vi "RearrangePoints.vi"() -> (2 "Iterations":i32)   [LabVIEW 2010]
panel:
  out "error out":errorcluster
  in  "error in (no error)":errorcluster
  in  "Parameters":T1={"number of planes"=4, "z step"=1.9999999999999998e-05, "pixel dwell time"=1.0000000000000001e-11, "z frequency"=10.0, "number of pixels"=100, "smooth points"=10, "smooth line"=10, "Sine\nSawtooth"=FALSE, "PointSorting"=0, "Sort Points"=FALSE, "X-pixels"=256.0, "Y-lines"=256.0} {"Y-lines" min=1 step=1; "X-pixels" min=1 step=1; "PointSorting" items=["No Difference", "Every Second Point", "Down / Up"]; "smooth line" min=1; "smooth points" min=1; "number of pixels" min=1; "z frequency" format="%_4g"; "number of planes" min=1}
  out "XYZ Point coordinates updated (pixels) Up":dbl[][](array[numeric])
  out "XYZ Point coordinates updated (pixels) Down":dbl[][](array[numeric])
  in  "XYZ Point coordinates (pixels)":dbl[][](array[numeric])
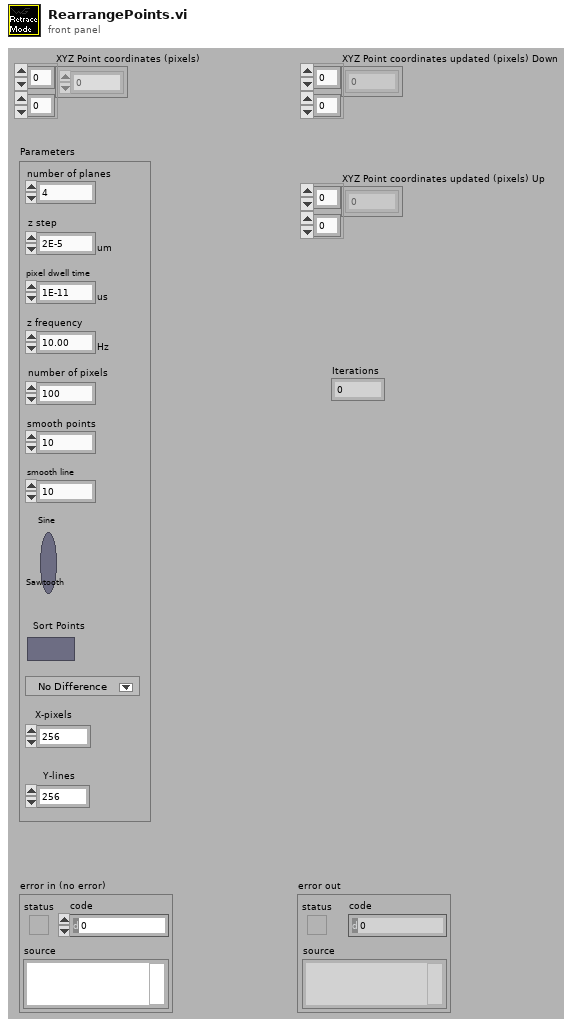
[diagram p1: front panel]
types:
  T1 = cluster{"number of planes":i32, "z step":dbl[unit], "pixel dwell time":dbl[unit], "z frequency":dbl[unit], "number of pixels":i32, "smooth points":i32, "smooth line":i32, "Sine\nSawtooth":bool, "PointSorting":u16, "Sort Points":bool, "X-pixels":sgl, "Y-lines":sgl}
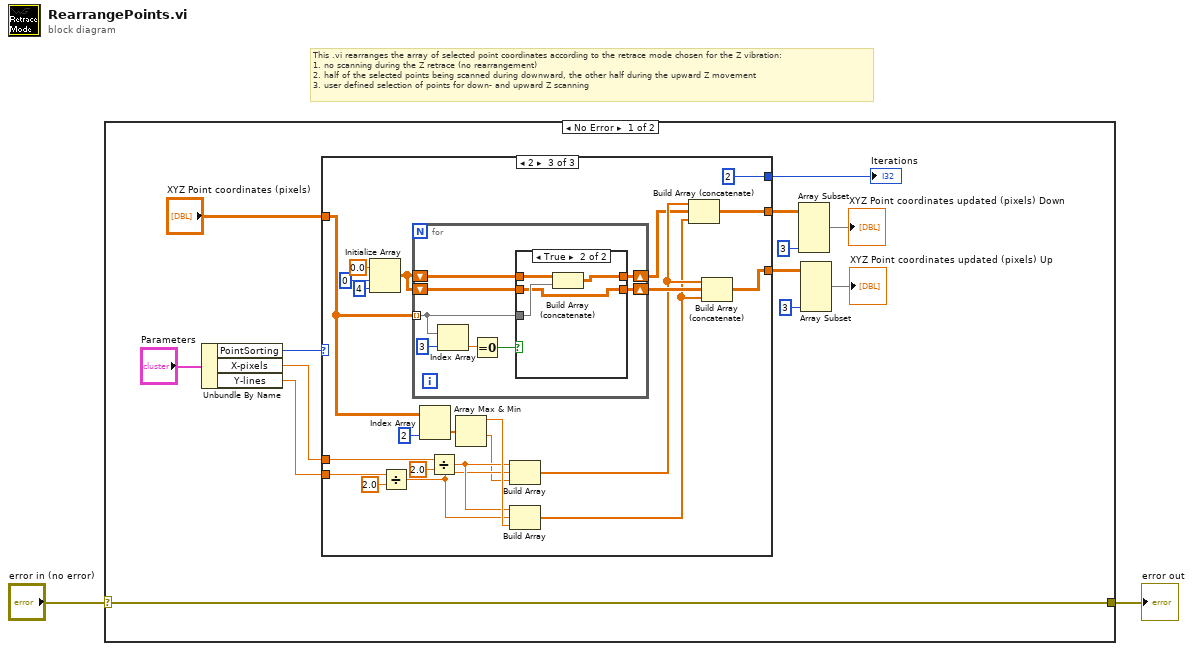
[diagram p0: block diagram]
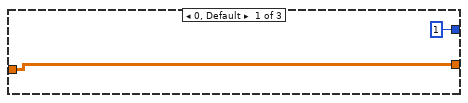
[diagram p2: hidden frame]
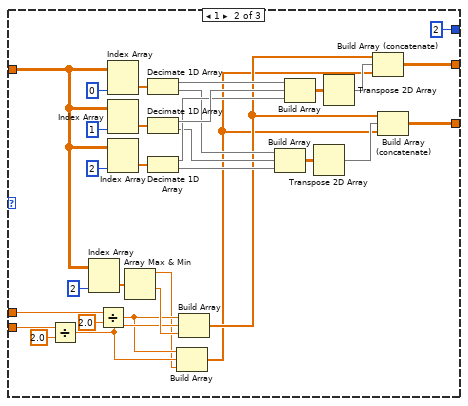
[diagram p3: hidden frame]
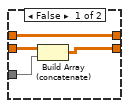
[diagram p4: hidden frame]
diagram:
  # "This .vi rearranges the array of selected point coordinates according to the retrace mode chosen for the Z vibration:\n1. no scanning during the Z retrace (no rearrangement)\n2. half of the selected points being scanned during downward, the other half during the upward Z movement\n3. user defined selection of points for down- and upward Z scanning"
  n1 = case shown="No Error" "error in (no error)" {
    selector: "error in (no error)" -> [w3 w88]
    tunnel: [w3 w88] -> w1
    frame No Error {
      n2 = Unbundle By Name("Parameters") -> ("PointSorting"=w6:u16, "X-pixels"=w5:sgl, "Y-lines"=w4:sgl)
      n3 = case shown="2" w6 {
        tunnel: "XYZ Point coordinates (pixels)" -> [w17 w23 w58]
        tunnel: w5 -> [_ w22 w60]
        tunnel: w4 -> [_ w21 w59]
        tunnel: [w17 w20 w57] -> w13
        tunnel: [_ w19 w53] -> w11
        tunnel: [1 2 2] -> w15
        frame 0, Default {
        }
        frame 1 {
          n4 = Divide(x=w21, y=2.0) -> (x/y=w28:dbl)
          n5 = Index Array(array=w23, index (col)=2 ("disabled index (col)")) -> (element=w32:dbl[])  [unwired: 1 in]
          n6 = Divide(x=w22, y=2.0) -> (x/y=w27:dbl)
          n7 = Index Array(array=w23, index (col)=0 ("disabled index (col)")) -> (element=w46:dbl[])  [unwired: 1 in]
          n8 = Index Array(array=w23, index (col)=1 ("disabled index (col)")) -> (element=w45:dbl[])  [unwired: 1 in]
          n9 = Index Array(array=w23, index (col)=2 ("disabled index (col)")) -> (element=w44:dbl[])  [unwired: 1 in]
          n10 = Array Max & Min(array=w32) -> (max value=w26:dbl, min value=w29:dbl)  [unwired: 2 out]
          n11 = Decimate 1D Array(w46) -> (w42:dbl[], w36:dbl[])
          n12 = Decimate 1D Array(w45) -> (w41:dbl[], w37:dbl[])
          n13 = Decimate 1D Array(w44) -> (w40:dbl[], w38:dbl[])
          n14 = Build Array(w27, w28, w26) -> (w24:dbl[])
          n15 = Build Array(w27, w28, w29) -> (w25:dbl[])
          n16 = Build Array(w36, w37, w38) -> (w39:dbl[][])
          n17 = Build Array(w42, w41, w40) -> (w43:dbl[][])
          n18 = Transpose 2D Array(2D array=w39) -> (transposed array=w34:dbl[][])
          n19 = Transpose 2D Array(2D array=w43) -> (transposed array=w35:dbl[][])
          n20 = Build Array (concatenate)(w25, w35, w24) -> (w20:dbl[][])
          n21 = Build Array (concatenate)(w25, w34, w24) -> (w19:dbl[][])
        }
        frame 2 {
          n22 = Initialize Array(0.0 ("element"), 0 ("dimension size"), 4 ("dimension size")) -> (w69:dbl[][])
          n23 = Divide(x=w59, y=2.0) -> (x/y=w66:dbl)
          n24 = for {
            tunnel: w58 -> [w76] mode=indexing
            shift-right: [w74] -> w52
            shift-left: w69 -> [w75]
            shift-right: [w72] -> w56
            shift-left: w69 -> [w73]
            n25 = Index Array(array=w76, index=3) -> (element=w78:dbl)
            n26 = Equal To 0?(x=w78) -> (x = 0?=w77:bool)
            n27 = case shown="True" w77 {
              tunnel: w76 -> [w80 w86]
              tunnel: w75 -> [w83 w87]
              tunnel: [w83 w85] -> w74
              tunnel: w73 -> [w82 w84]
              tunnel: [w81 w84] -> w72
              frame False {
                n28 = Build Array (concatenate)(w82, w80) -> (w81:dbl[][])
              }
              frame True {
                n29 = Build Array (concatenate)(w87, w86) -> (w85:dbl[][])
              }
            }
          }
          n30 = Index Array(array=w58, index (col)=2 ("disabled index (col)")) -> (element=w62:dbl[])  [unwired: 1 in]
          n31 = Divide(x=w60, y=2.0) -> (x/y=w67:dbl)
          n32 = Array Max & Min(array=w62) -> (max value=w68:dbl, min value=w65:dbl)  [unwired: 2 out]
          n33 = Build Array(w67, w66, w65) -> (w55:dbl[])
          n34 = Build Array(w67, w66, w68) -> (w54:dbl[])
          n35 = Build Array (concatenate)(w55, w52, w54) -> (w57:dbl[][])
          n36 = Build Array (concatenate)(w55, w56, w54) -> (w53:dbl[][])
        }
      }
      "Iterations" <- w15
      n37 = Array Subset(array=w13, length (col)=3 ("length")) -> (→"XYZ Point coordinates updated (pixels) Down":dbl[][])  [unwired: 3 in]
      n38 = Array Subset(array=w11, length (col)=3 ("length")) -> (→"XYZ Point coordinates updated (pixels) Up":dbl[][])  [unwired: 3 in]
    }
    frame Error {
    }
  }
  "error out" <- w1
